vi "GeneratePlaneEquation.vi"(8 "Error In":errorcluster, 11 "Three  points":dbl[][](array[numeric])) -> (0 "Error Out":errorcluster, 1 "Equation":string, 2 "D":dbl, 3 "NormalVector":dbl[](array[numeric]))   [LabVIEW 2019]
uses:
  <vilib>/Analysis/baseanly.llb/Real Dot Product.vi
  <vilib>/Analysis/NI_AALBase.lvlib
panel:
  out "Counter2":i32
  out "Counter":i32
  out "V2":dbl[](array[numeric])
  out "V1":dbl[](array[numeric])
  # "Ax + By + Cz = <A,B,C> . <X_0,Y_0,Z_0> = D"
  # "Nx"
  # "Ny"
  # "Nz"
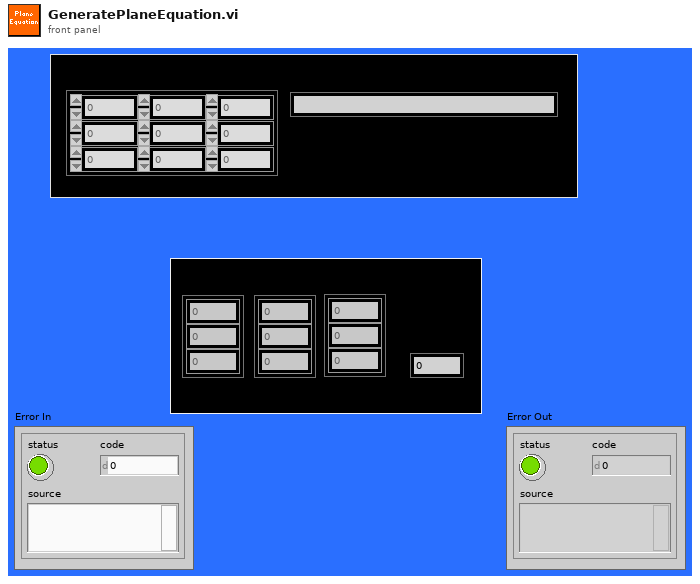
[diagram p1: front panel]
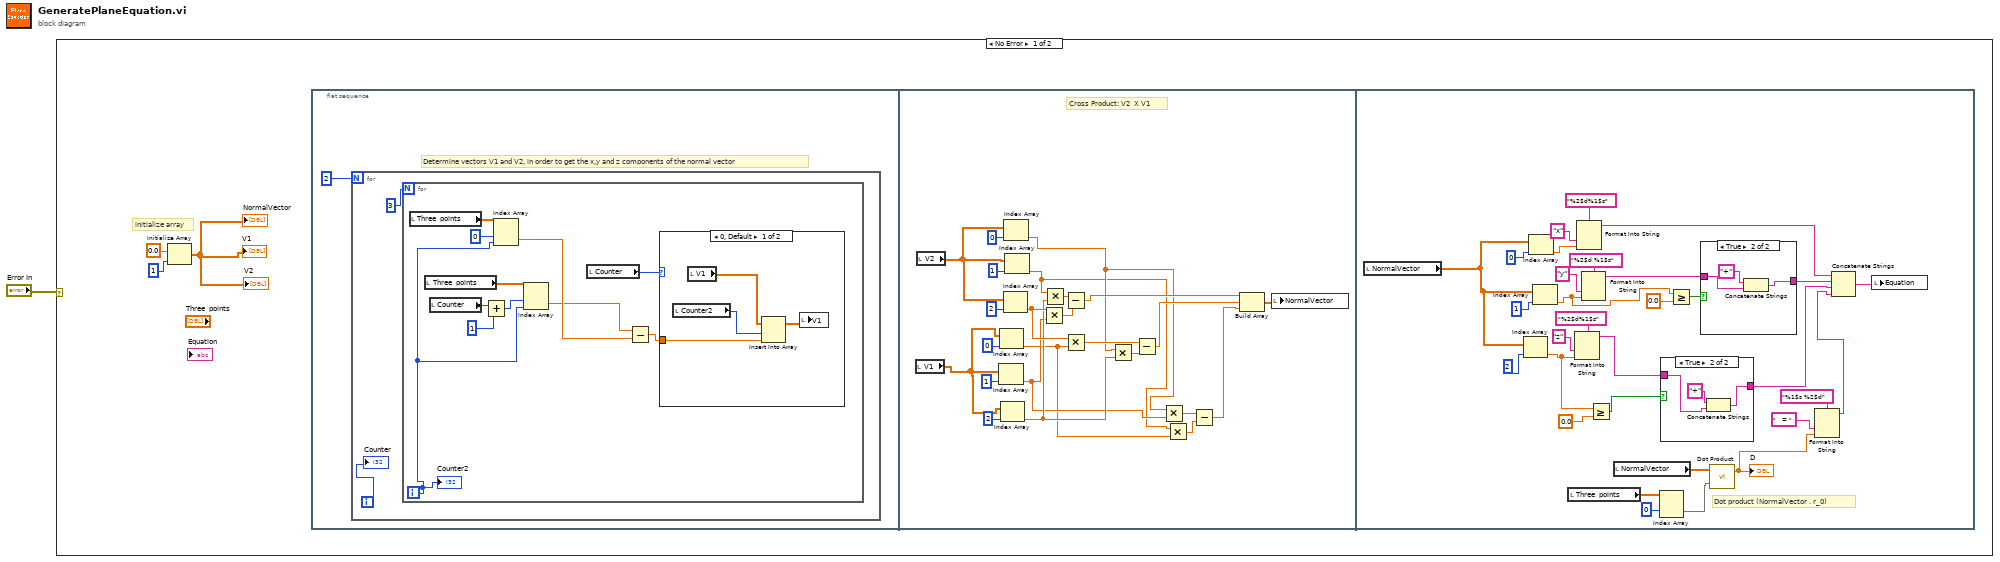
[diagram p0: block diagram]
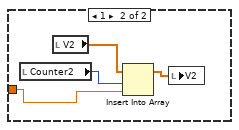
[diagram p2: hidden frame]
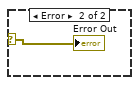
[diagram p5: hidden frame]
diagram:
  n1 = case shown="No Error" "Error In" {
    selector: "Error In" -> [_ w90]
    frame No Error {
      # "initialize array"
      n2 = Initialize Array(0.0 ("element"), 1 ("dimension size")) -> (→"NormalVector" →"V1" →"V2":dbl[])
      n3 = flat-sequence {
        frame #0 {
          # "Determine vectors V1 and V2, in order to get the x,y and z components of the normal vector"
          n4 = for {
            N: 2 -> [_]
            i -> [w6]
            n5 = for {
              N: 3 -> [_]
              i -> [w10]
              n6 = local read "Three  points"() -> (w18:dbl[][])
              n7 = local read "Three  points"() -> (w15:dbl[][])
              n8 = local read "Counter"() -> (w14:i32)
              n9 = Add(x=w14, y=1) -> (x+y=w12:i32)
              n10 = Index Array(array=w18, index (row)=0, index (col)=w10) -> (element=w11:dbl)
              n11 = Index Array(array=w15, index (row)=w12, index (col)=w10) -> (element=w8:dbl)
              n12 = local read "Counter"() -> (w16:i32)
              n13 = Subtract(x=w8, y=w11) -> (x-y=w9:dbl)
              n14 = case shown="0, Default" w16 {
                tunnel: w9 -> [w20 w23]
                frame 0, Default {
                  n15 = local read "Counter2"() -> (w19:i32)
                  n16 = local read "V1"() -> (w21:dbl[])
                  n17 = Insert Into Array(array=w21, index=w19, new element=w20) -> (w22:dbl[])
                  n18 = local write "V1"(w22) -> ()
                }
                frame 1 {
                  n19 = local read "Counter2"() -> (w24:i32)
                  n20 = local read "V2"() -> (w25:dbl[])
                  n21 = Insert Into Array(array=w25, index=w24, new element=w23) -> (w26:dbl[])
                  n22 = local write "V2"(w26) -> ()
                }
              }
              "Counter2" <- w10
            }
            "Counter" <- w6
          }
        }
        frame #1 {
          # "Cross Product: V2  X V1"
          n23 = local read "V1"() -> (w46:dbl[])
          n24 = local read "V2"() -> (w50:dbl[])
          n25 = Index Array(array=w46, index=1) -> (element=w31:dbl)
          n26 = Index Array(array=w46, index=0) -> (element=w29:dbl)
          n27 = Index Array(array=w46, index=2) -> (element=w36:dbl)
          n28 = Index Array(array=w50, index=2) -> (element=w39:dbl)
          n29 = Index Array(array=w50, index=0) -> (element=w32:dbl)
          n30 = Index Array(array=w50, index=1) -> (element=w30:dbl)
          n31 = Multiply(x=w39, y=w31) -> (x*y=w41:dbl)
          n32 = Multiply(x=w30, y=w36) -> (x*y=w42:dbl)
          n33 = Subtract(x=w42, y=w41) -> (x-y=w40:dbl)
          n34 = Multiply(x=w39, y=w29) -> (x*y=w38:dbl)
          n35 = Multiply(x=w32, y=w36) -> (x*y=w37:dbl)
          n36 = Subtract(x=w38, y=w37) -> (x-y=w35:dbl)
          n37 = Multiply(x=w32, y=w31) -> (x*y=w34:dbl)
          n38 = Multiply(x=w30, y=w29) -> (x*y=w33:dbl)
          n39 = Subtract(x=w34, y=w33) -> (x-y=w28:dbl)
          n40 = Build Array(w40, w35, w28) -> (w27:dbl[])
          n41 = local write "NormalVector"(w27) -> ()
        }
        frame #2 {
          # "Dot product (NormalVector . r_0)"
          n42 = local read "NormalVector"() -> (w74:dbl[])
          n43 = Index Array(array=w74, index=2) -> (element=w58:dbl)
          n44 = Index Array(array=w74, index=0) -> (element=w55:dbl)
          n45 = Index Array(array=w74, index=1) -> (element=w59:dbl)
          n46 = local read "Three  points"() -> (w80:dbl[][])
          n47 = Format Into String(format string="%2$d%1$s", "z" ("initial string"), w58) -> (resulting string=w68:string)  [unwired: 2 in, 1 out]
          n48 = Format Into String(format string="%2$d%1$s", "x" ("initial string"), w55) -> (resulting string=w67:string)  [unwired: 2 in, 1 out]
          n49 = Format Into String(format string="%2$d %1$s", "y" ("initial string"), w59) -> (resulting string=w69:string)  [unwired: 2 in, 1 out]
          n50 = Greater Or Equal?(x=w58, y=0.0) -> (x >= y?=w71:bool)
          n51 = local read "NormalVector"() -> (w81:dbl[])
          n52 = Index Array(array=w80, index (row)=0) -> (element=w78:dbl[])  [unwired: 1 in]
          n53 = case shown="True" w71 {
            tunnel: w68 -> [w82 w84]
            tunnel: [w82 w83] -> w65
            frame False {
            }
            frame True {
              n54 = Concatenate Strings("+" ("string"), w84) -> (w83:string)
            }
          }
          n55 = Greater Or Equal?(x=w59, y=0.0) -> (x >= y?=w72:bool)
          n56 = case shown="True" w72 {
            tunnel: w69 -> [w86 w88]
            tunnel: [w86 w87] -> w66
            frame False {
            }
            frame True {
              n57 = Concatenate Strings("+" ("string"), w88) -> (w87:string)
            }
          }
          n58 = call-poly <vilib>:"Dot Product.vi"("Y Vector"=w78, "X Vector"=w81) -> ("X * Y"=w51:dbl)  [unwired: 1 out]
          "D" <- w51
          n59 = Format Into String(format string="%1$s %2$d", "   = " ("initial string"), w51) -> (resulting string=w64:string)  [unwired: 2 in, 1 out]
          n60 = Concatenate Strings(w67, w66, w65, w64) -> (w63:string)
          n61 = local write "Equation"(w63) -> ()
        }
      }
    }
    frame Error {
      "Error Out" <- w90
    }
  }
